vi "Validate Configuration.vi"(8 "error in":errorcluster, 11 "SystemConfigRepo in":refnum<class "SystemConfigRepo.lvclass">) -> (0 "error out":errorcluster, 3 "SystemConfigRepo out":refnum<class "SystemConfigRepo.lvclass">)   [LabVIEW 2013, in "PL Framework Configuration Tool.lvlib" / "SystemConfigRepo.lvclass"]
uses:
  SystemConfigRepo.lvclass
  SystemConfigRepo.lvclass/SystemConfigRepo.ctl
  Framework Configuration Classes/system configuration/PL_System Configuration.lvclass
  Framework Configuration Classes/target configuration/PL_Target Configuration.lvclass
  <vilib>/NI/Module Execution Interface/Engine Configuration/engine configuration.lvclass
  <vilib>/NI/Tag Bus Module Framework/module configuration/TBM module configuration.lvclass
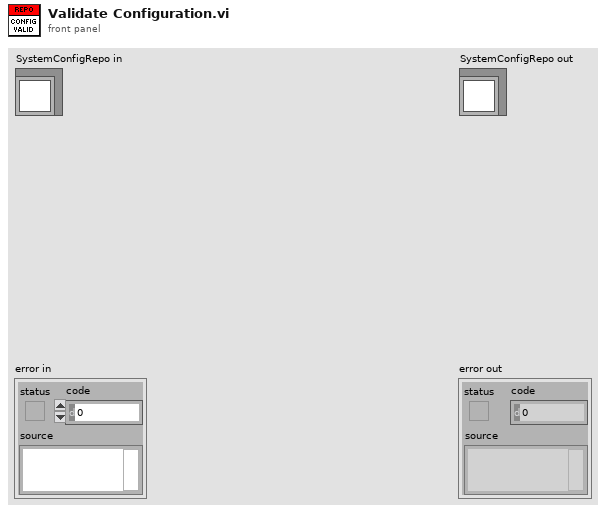
[diagram p1: front panel]
types:
  T1 = typedef "PLConfigurationSerializer.lvlib/targets cluster.ctl" = cluster{"Target Configuration":refnum<class "PL_Target Configuration.lvclass">, "engines":T2[]}
  T2 = typedef "PLConfigurationSerializer.lvlib/engines cluster.ctl" = cluster{"engine configuration":refnum<class "engine configuration.lvclass">, "modules":refnum<class "TBM module configuration.lvclass">[]}
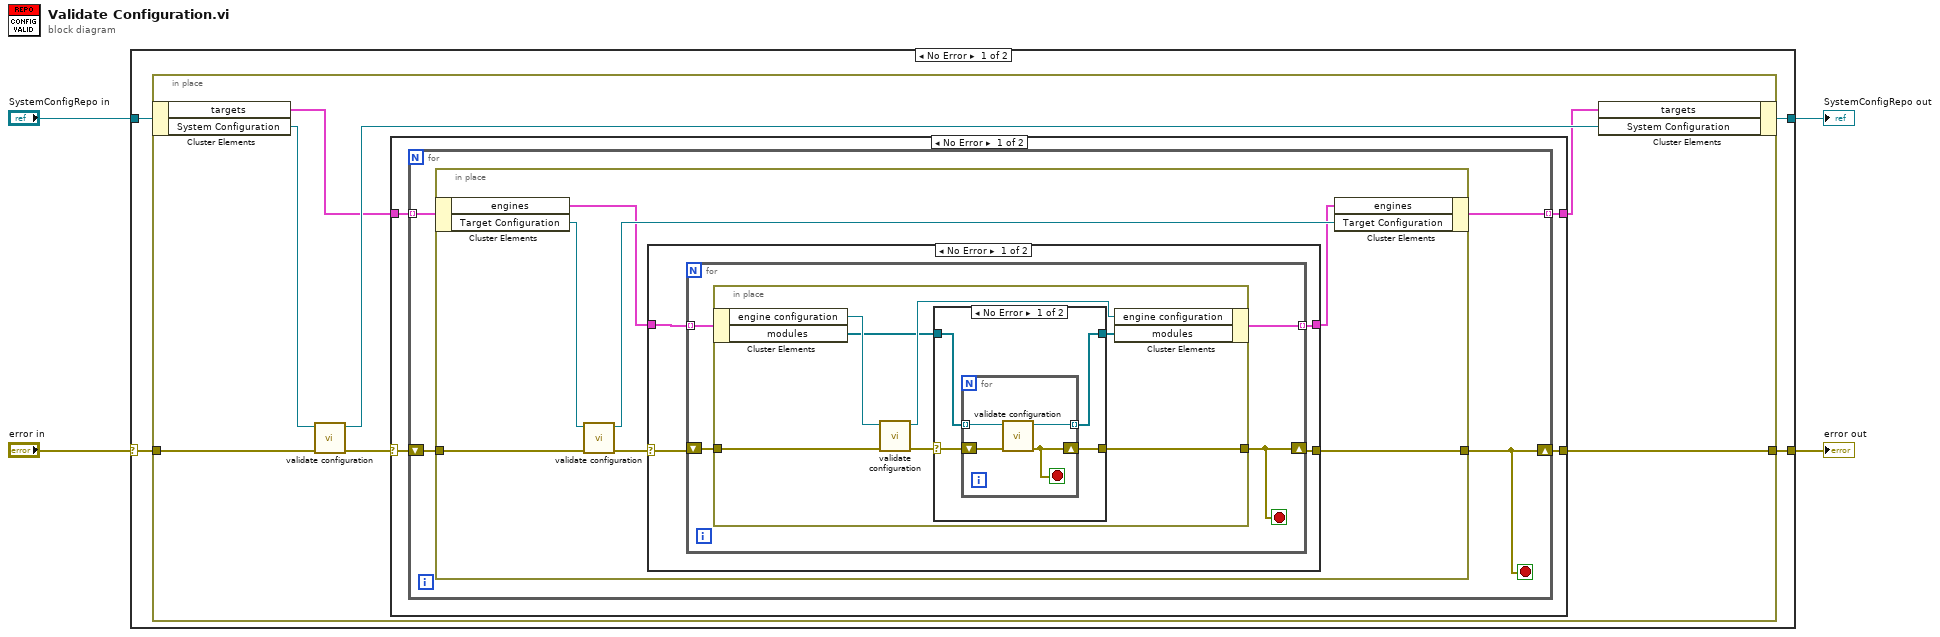
[diagram p0: block diagram]
diagram:
  n1 = case shown="No Error" "error in" {
    selector: "error in" -> [w6 w61]
    tunnel: [w5 w61] -> w3
    tunnel: [w7 w60] -> w1
    tunnel: "SystemConfigRepo in" -> [w8 w60]
    frame No Error {
      n2 = in-place {
        in-place-border: w6 -> [w15]
        in-place-border: [w11] -> w5
        n3 = in-place-cluster #1(w8) -> ("targets"=w12:T1[], "System Configuration"=w14:refnum<class "PL_System Configuration.lvclass">)
        n4 = call-dynamic "validate configuration.vi"("error in"=w15, "configuration in"=w14) -> ("error out"=w9:errorcluster, "configuration out"=w13:refnum<class "PL_System Configuration.lvclass">)  [unwired: 8 in]
        n5 = case shown="No Error" w9 {
          selector: w9 -> [w16 w58]
          tunnel: w12 -> [w19 w59]
          tunnel: [w18 w58] -> w11
          tunnel: [w17 w59] -> w10
          frame No Error {
            n6 = for {
              tunnel: w19 -> [w23] mode=indexing
              shift-right: [w20] -> w18
              shift-left: w16 -> [w21]
              tunnel: [w22] -> w17 mode=indexing
              stop <- w20 stop-if-true
              n7 = in-place {
                in-place-border: w21 -> [w29]
                in-place-border: [w25] -> w20
                n8 = in-place-cluster #2(w23) -> ("engines"=w27:T2[], "Target Configuration"=w30:refnum<class "PL_Target Configuration.lvclass">)
                n9 = call-dynamic "validate configuration.vi"("error in"=w29, "configuration in"=w30) -> ("error out"=w24:errorcluster, "configuration out"=w28:refnum<class "PL_Target Configuration.lvclass">)  [unwired: 8 in]
                n10 = case shown="No Error" w24 {
                  selector: w24 -> [w31 w56]
                  tunnel: w27 -> [w34 w57]
                  tunnel: [w33 w57] -> w26
                  tunnel: [w32 w56] -> w25
                  frame No Error {
                    n11 = for {
                      tunnel: w34 -> [w38] mode=indexing
                      tunnel: [w37] -> w33 mode=indexing
                      shift-right: [w35] -> w32
                      shift-left: w31 -> [w36]
                      stop <- w35 stop-if-true
                      n12 = in-place {
                        in-place-border: w36 -> [w43]
                        in-place-border: [w42] -> w35
                        n13 = in-place-cluster #3(w38) -> ("engine configuration"=w45:refnum<class "engine configuration.lvclass">, "modules"=w41:refnum<class "TBM module configuration.lvclass">[])
                        n14 = call-dynamic "validate configuration.vi"("error in"=w43, "engine configuration in"=w45) -> ("error out"=w39:errorcluster, "engine configuration out"=w44:refnum<class "engine configuration.lvclass">)  [unwired: 8 in]
                        n15 = case shown="No Error" w39 {
                          selector: w39 -> [w46 w54]
                          tunnel: [w49 w54] -> w42
                          tunnel: w41 -> [w48 w55]
                          tunnel: [w47 w55] -> w40
                          frame No Error {
                            n16 = for {
                              shift-right: [w50] -> w49
                              shift-left: w46 -> [w53]
                              tunnel: w48 -> [w52] mode=indexing
                              tunnel: [w51] -> w47 mode=indexing
                              stop <- w50 stop-if-true
                              n17 = call-dynamic "validate configuration.vi"("error in"=w53, "configuration in"=w52) -> ("error out"=w50:errorcluster, "configuration out"=w51:refnum<class "TBM module configuration.lvclass">)  [unwired: 8 in]
                            }
                          }
                          frame Error {
                          }
                        }
                        n18 = in-place-cluster #3("engine configuration"=w44, "modules"=w40) -> (w37:T2)
                      }
                    }
                  }
                  frame Error {
                  }
                }
                n19 = in-place-cluster #2("engines"=w26, "Target Configuration"=w28) -> (w22:T1)
              }
            }
          }
          frame Error {
          }
        }
        n20 = in-place-cluster #1("targets"=w10, "System Configuration"=w13) -> (w7:refnum<class "SystemConfigRepo.lvclass">)
      }
    }
    frame Error {
    }
  }
  "error out" <- w3
  "SystemConfigRepo out" <- w1
